vi "Alternate-triggering-test.vi"() -> ()   [LabVIEW 2016]
uses:
  <vilib>/Platform/TimedLoop/XDataNode/timing_clust.ctl
  <vilib>/Platform/TimedLoop/XDataNode/nitl_modes.ctl
  <vilib>/Platform/TimedLoop/XDataNode/wakeup.ctl
  <vilib>/xnet/xnet.llb/XNET Write (Signal Single-point).vi
  <vilib>/Platform/TimedLoop/XDataNode/XDataNode.xnode
  <vilib>/Platform/TimedLoop/XDataNode/XDNodeRunTimeDep.lvlib
panel:
  in  "Trig count 2":dbl
  in  "Trig count 1":dbl
  in  "Plant to trigg":u16(ring) items=["Plant 1"=1, "Plant 2"=2]
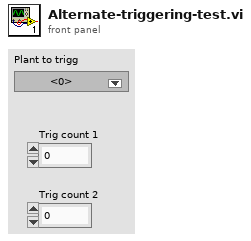
[diagram p1: front panel]
types:
  T1 = typedef "XDNodeRunTimeDep.lvlib/timing_clust.ctl" = cluster{"Expected End [f-1]":u64, "Actual End [f-1]":u64, "Finished Late? [f-1]":bool, "Expected End [i-1]":u64, "Actual End [i-1]":u64, "Finished Late? [i-1]":bool, "Expected Start [i]":u64, "Actual Start [i]":u64, "Expected Start [f]":u64, "Actual Start [f]":u64, "Source Name":string, "Structure Name":string, "Period":i64, "Deadline":i64, "Offset":i64, "Start":i64, "Priority":i32, "Timeout":i32, "Mode":T2, "Wakeup Reason":T3, "Error":errorcluster, "Source Type":string, "Secondary Source Type":string, "Global End Time":u64, "Global Start Time":u64, "Frame Duration":u64, "Iteration Duration":u64, "Assigned CPU":i32, "I/O Scan Engine Mode":u32}
  T2 = typedef "XDNodeRunTimeDep.lvlib/nitl_modes.ctl" = enum32{"No Change", "Process missed periods, maintain original phase", "Discard missed periods, maintain original phase", "Process missed periods, ignore original phase", "Discard missed periods, ignore original phase"}
  T3 = typedef "XDNodeRunTimeDep.lvlib/wakeup.ctl" = enum32{"Normal", "Aborted", "Asynchronous wakeup", "Timing source error", "Timed loop error", "Timeout"}
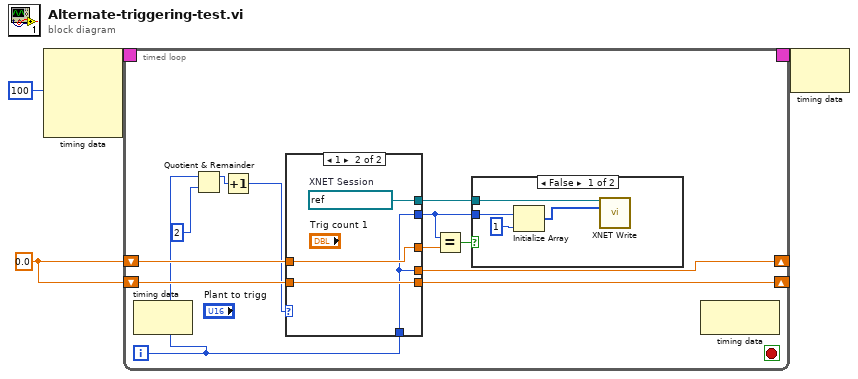
[diagram p0: block diagram]
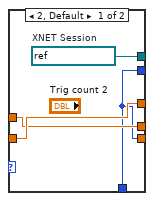
[diagram p3: hidden frame]
diagram:
  w1 = 0.0 ("Trig count 2")
  n1 = node-c288(i64 100 ("Period")) -> (w4:T1)  [unwired: 3 in]
  n2 = timed-loop {
    timing: w4 -> [_]
    timing-out: [_] -> w3
    shift-right: [w10] -> _
    shift-left: w1 -> [w16]
    shift-right: [w9] -> _
    shift-left: w1 -> [w11]
    i -> [w8]
    stop <- _ stop-if-true
    n3 = node-c288() -> ()  [unwired: 1 in, 1 out]
    n4 = Quotient & Remainder(x=w8, y=2) -> (x-y*floor(x/y)=w6:i32)  [unwired: 1 out]
    n5 = Increment(x=w6) -> (x+1=w5:i32)
    n6 = case shown="1" w5 {
      tunnel: [w24 w28] -> w12
      tunnel: w16 -> [w22 w27]
      tunnel: [w21 w25] -> w13
      tunnel: [w23 w27] -> w14
      tunnel: w11 -> [w23 w26]
      tunnel: [w22 w25] -> w10
      tunnel: [w21 w26] -> w9
      tunnel: w8 -> [w21 w25]
      frame 2, Default {
        w24 = refnum<k21> "Plant2_trig"  # XNET Session
      }
      frame 1 {
        w28 = refnum<k21> "Plant1_trig"  # XNET Session
      }
    }
    n7 = Equal?(x=w13, y=w14) -> (x = y?=w15:bool)
    n8 = case shown="False" w15 {
      tunnel: w12 -> [w20 _]
      tunnel: w13 -> [w17 _]
      frame False {
        n9 = Initialize Array(w17, 1 ("dimension size")) -> (w18:i32[])
        n10 = call-poly <vilib>:"XNET Write.vi"("session in"=w20, "data"=w18) -> ()  [unwired: 12 in, 2 out]
      }
      frame True {
      }
    }
    n11 = node-c288() -> ()  [unwired: 1 in, 1 out]
  }
  n12 = node-c288(w3) -> ()  [unwired: 1 out]
